vi "destroyUserEvents.vi"(8 "error in (no error)":errorcluster, 11 "UserEvents in":refnum<class "UserEvents.lvclass">) -> (0 "error out":errorcluster, 3 "UserEvents out":refnum<class "UserEvents.lvclass">)   [LabVIEW 2016, in "UserEvents.lvclass"]
uses:
  UserEvents.lvclass
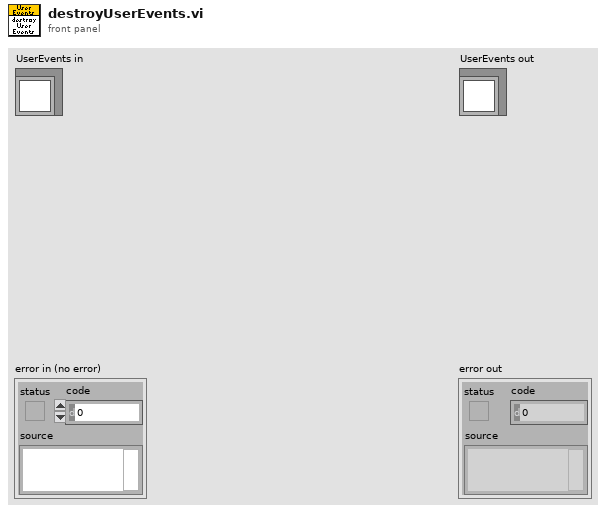
[diagram p1: front panel]
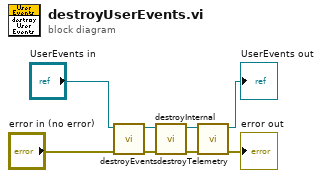
[diagram p0: block diagram]
diagram:
  n1 = call "destroyEvents.vi"("error in (no error)"="error in (no error)", "UserEvents in"="UserEvents in") -> ("error out"=w2:errorcluster, "UserEvents out"=w5:refnum<class "UserEvents.lvclass">)  [unwired: 8 in]
  n2 = call "destroyInternal.vi"("error in (no error)"=w2, "UserEvents in"=w5) -> ("error out"=w1:errorcluster, "UserEvents out"=w4:refnum<class "UserEvents.lvclass">)  [unwired: 8 in]
  n3 = call "destroyTelemetry.vi"("error in (no error)"=w1, "UserEvents in"=w4) -> ("error out"=→"error out":errorcluster, "UserEvents out"=→"UserEvents out":refnum<class "UserEvents.lvclass">)  [unwired: 8 in]
